vi "Is Default.vi"(11 "Subscription Token In":refnum<class "Subscription Token.lvclass">) -> (2 "is default":bool, 3 "Subscription Token Out":refnum<class "Subscription Token.lvclass">)   [LabVIEW 2016, in "Data Broadcasting.lvlib" / "Subscription Token.lvclass"]
doc: "Checks a Subscription Token against its default instance. This method can be used to verify that a token carries a non-default configuration. However, it cannot guarantee that the configuration is valid. The configuration may hold an NQR for a Broadcaster that has stopped.\n\n\n-------------\nCopyright (c) 2013, Staab Engineering, a Texas Limited Liability Company\nAll rights reserved.\n\nRedistribution and use in source and binary forms, with or without modification, are permitted provided that the following conditions are met:\n\n1. Redistributions of source code must retain the above copyright notice, this list of conditions and the following disclaimer.\n2. Redistributions in binary form must reproduce the above copyright notice, this list of conditions and the following disclaimer in the documentation and/or other materials provided with the distribution.\n\nTHIS SOFTWARE IS PROVIDED BY THE COPYRIGHT HOLDERS AND CONTRIBUTORS \"AS IS\" AND ANY EXPRESS OR IMPLIED WARRANTIES, INCLUDING, BUT NOT LIMITED TO, THE IMPLIED WARRANTIES OF MERCHANTABILITY AND FITNESS FOR A PARTICULAR PURPOSE ARE DISCLAIMED. IN NO EVENT SHALL THE COPYRIGHT HOLDER OR CONTRIBUTORS BE LIABLE FOR ANY DIRECT, INDIRECT, INCIDENTAL, SPECIAL, EXEMPLARY, OR CONSEQUENTIAL DAMAGES (INCLUDING, BUT NOT LIMITED TO, PROCUREMENT OF SUBSTITUTE GOODS OR SERVICES; LOSS OF USE, DATA, OR PROFITS; OR BUSINESS INTERRUPTION) HOWEVER CAUSED AND ON ANY THEORY OF LIABILITY, WHETHER IN CONTRACT, STRICT LIABILITY, OR TORT (INCLUDING NEGLIGENCE OR OTHERWISE) ARISING IN ANY WAY OUT OF THE USE OF THIS SOFTWARE, EVEN IF ADVISED OF THE POSSIBILITY OF SUCH DAMAGE."
uses:
  <userlib>/_Frameworks/Staab/AF Data Broadcasting/Data Broadcasting/Subscription Token/Subscription Token.lvclass
  <userlib>/_Frameworks/Staab/AF Data Broadcasting/Data Broadcasting/Registration Msg/Registration Msg.lvclass
  <userlib>/_Frameworks/Staab/AF Data Broadcasting/Data Broadcasting/Unregistration Msg/Unregistration Msg.lvclass
  <userlib>/_Frameworks/Staab/AF Data Broadcasting/Data Broadcasting/Subscription Token/Subscription Token.lvclass/Subscription Token.ctl
  <vilib>/ActorFramework/Message Enqueuer/Message Enqueuer.lvclass
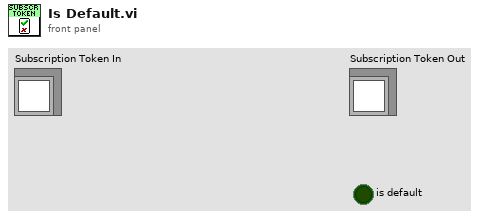
[diagram p1: front panel]
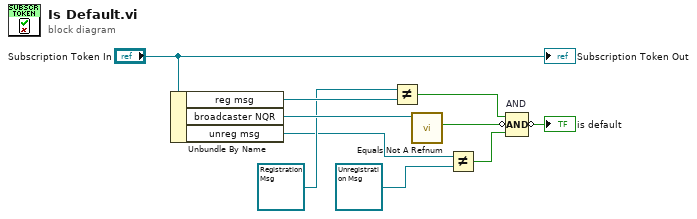
[diagram p0: block diagram]
diagram:
  n1 = Unbundle By Name("Subscription Token In") -> ("reg msg"=w6:refnum<class "Registration Msg.lvclass">, "broadcaster NQR"=w8:refnum<class "Message Enqueuer.lvclass">, "unreg msg"=w4:refnum<class "Unregistration Msg.lvclass">)
  n2 = Not Equal?(x=refnum<class "Registration Msg.lvclass"> refnum ("af_Data Broadcasting.lvlib:Subscription Msg.lvclass"), y=w6) -> (x != y?=w2:bool)
  n3 = call <vilib>:"Equals Not A Refnum.vi"("Message Enqueuer"=w8) -> ("Not a refnum?"=w7:bool)  [unwired: 10 in]
  n4 = Not Equal?(x=w4, y=refnum<class "Unregistration Msg.lvclass"> refnum ("af_Data Broadcasting.lvlib:Unsubscription Msg.lvclass")) -> (x != y?=w1:bool)
  n5 = Compound Arithmetic op=AND "AND"(w2, invert w7, w1) -> (invert →"is default":bool)
  "Subscription Token Out" <- "Subscription Token In"
